vi "Serialize.vi"(0 "object in":refnum<class "JSONJKI.lvclass">, 2 "outputs":variant[](array[variant]), 5 "error in (no error)":errorcluster) -> (14 "object out":refnum<class "JSONJKI.lvclass">, 16 "JSON":string, 19 "error out":errorcluster)   [LabVIEW 2018, in "JSONJKI.lvclass"]
uses:
  JSONJKI.lvclass
  <vilib>/addons/_JKI.lib/Serialization/JSON/Serializer/JSON Serializer/JSON Serializer.lvclass
  <vilib>/addons/_JKI.lib/Serialization/JSON/JKI JSON Serialization.lvlib
  <vilib>/Utility/Data Type/NI_Data Type.lvlib
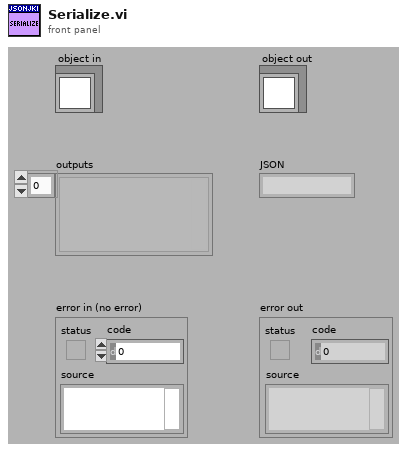
[diagram p1: front panel]
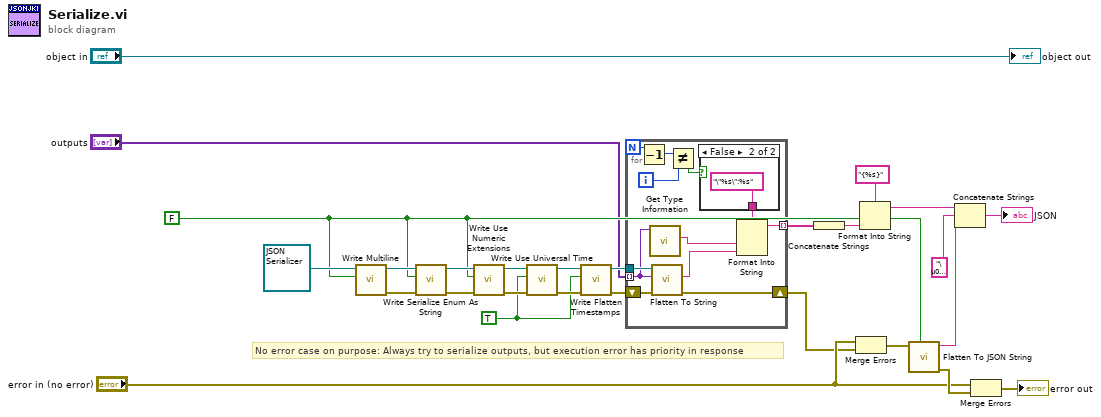
[diagram p0: block diagram]
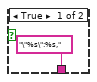
[diagram p2: hidden frame]
diagram:
  w9 = TRUE ("Convert Timestamps")
  w8 = FALSE ("Multiline (T)")
  # "No error case on purpose: Always try to serialize outputs, but execution error has priority in response"
  n1 = call-dynamic "Write Multiline.vi"("Multiline"=w8, "JSON Serializer in"=refnum<class "JSON Serializer.lvclass"> refnum) -> ("error out"=w18:errorcluster, "JSON Serializer out"=w17:refnum<class "JSON Serializer.lvclass">)  [unwired: 8 in]
  n2 = call-dynamic "Write Serialize Enum As String.vi"("error in (no error)"=w18, "Enums As String"=w8, "JSON Serializer in"=w17) -> ("error out"=w19:errorcluster, "JSON Serializer out"=w20:refnum<class "JSON Serializer.lvclass">)  [unwired: 7 in]
  n3 = call-dynamic "Write Use Numeric Extensions.vi"("error in (no error)"=w19, "Numeric Extensions"=w8, "JSON Serializer in"=w20) -> ("error out"=w13:errorcluster, "JSON Serializer out"=w12:refnum<class "JSON Serializer.lvclass">)  [unwired: 7 in]
  n4 = call-dynamic "Write Use Universal Time.vi"("error in (no error)"=w13, "Universal Time"=w9, "JSON Serializer in"=w12) -> ("error out"=w14:errorcluster, "JSON Serializer out"=w10:refnum<class "JSON Serializer.lvclass">)  [unwired: 7 in]
  n5 = call-dynamic "Write Flatten Timestamps.vi"("error in (no error)"=w14, "Convert Timestamps"=w9, "JSON Serializer in"=w10) -> ("error out"=w15:errorcluster, "JSON Serializer out"=w16:refnum<class "JSON Serializer.lvclass">)  [unwired: 7 in]
  n6 = for {
    N -> [w32]
    tunnel: w16 -> [w38]
    tunnel: "outputs" -> [w37] mode=indexing
    shift-right: [w28] -> w1
    shift-left: w15 -> [w39]
    tunnel: [w33] -> w21 mode=indexing
    i -> [w30]
    n7 = Decrement(x=w32) -> (x-1=w31:i32)
    n8 = call <vilib>:"Get Type Information.vi"("Variant"=w37) -> ("Name"=w35:string)  [unwired: 6 in, 4 out]
    n9 = call-dynamic "Flatten To String.vi"("error in (no error)"=w39, "Variant"=w37, "JSON Serializer in"=w38) -> ("error out"=w28:errorcluster, "String"=w34:string)  [unwired: 6 in, 1 out]
    n10 = Not Equal?(x=w31, y=w30) -> (x != y?=w29:bool)
    n11 = case shown="False" w29 {
      tunnel: ["\"%s\":%s," ("format string") "\"%s\":%s" ("format string")] -> w36
      frame True {
      }
      frame False {
      }
    }
    n12 = Format Into String(format string=w36, w35, w34) -> (resulting string=w33:string)  [unwired: 2 in, 1 out]
  }
  n13 = Concatenate Strings(w21) -> (w23:string)
  n14 = Merge Errors("error in (no error)", w1) -> (w6:errorcluster)
  n15 = Format Into String(format string="{%s}", w23) -> (resulting string=w25:string)  [unwired: 2 in, 1 out]
  n16 = call <vilib>:"Flatten To JSON String.vi"("Multiline (T)"=w8, "Variant"=w6) -> ("error out"=w5:errorcluster, "JSON String"=w24:string)  [unwired: 8 in]
  n17 = Concatenate Strings(w25, "\u0017" ("Delimiter 3"), w24) -> (→"JSON":string)
  n18 = Merge Errors("error in (no error)", w5) -> (→"error out":errorcluster)
  "object out" <- "object in"
